vi "RHRT-IGVC-2013.vi"() -> ()   [LabVIEW 2012]
doc: "This the Rose-Hulman Robotics Tream IGVC compatition Code\nexample demonstrates the control of an autonomous robot through multiple asynchronous processes, modeled by VIs, that communicate with each other using shared variables. This example also shows an obstacle avoidance algorithm that the simulated robot uses as it navigates. The application includes the following processes:\n\n1. LIDAR Loop (\"Sense\")--Uses LabVIEW dataflow programming to generate simulated sensor data based on the position of the robot and any obstacles in the environment.\n\n2. Operator Loop (\"Think\")--Uses a state machine to control the movement of the robot according to commands from the user. When the robot follows a path without joystick or keyboard control, this process controls the attitude of the autonomous robot using a Vector Field Histogram (VFH) algorithm to avoid obstacles.\n\n3. Motor Loop (\"Act\")--Uses a Control and Simulation Loop, from the Control Design and Simulation Module, to create a model of the robot, simulate its dynamic behavior, and show the control loops and attitude observers."
uses:
  <vilib>/robotics/Controls/Compass Indicator/Compass Indicator.xctl
  <vilib>/Platform/TimedLoop/XDataNode/timing_clust.ctl
  <vilib>/Platform/TimedLoop/XDataNode/nitl_modes.ctl
  <vilib>/Platform/TimedLoop/XDataNode/wakeup.ctl
  <vilib>/Platform/TimedLoop/XDataNode/XDataNode.xnode
  <vilib>/Platform/TimedLoop/XDataNode/XDNodeRunTimeDep.lvlib
panel:
  out "Robot Model":u16
  in  "Robot Model:":T1(ring)
  out "Error":bool
  out "OK":bool
  in  "HUD 2":enum32{"GPS", "LIDAR", "IMU", "Occupancy Grid"}(tab)
  out "Health":u8(slide) scale=0.0..12.0
  out "XY Graph 2":cluster{dbl[], dbl[]}(graph)
  out "Data Aquired 2":picture
  out "Digree 2":dbl=16.3201904296875 caption="Digree"
  out "Compass Indicator 2":dbl(xcontrol)=16.3201904296875
  out "Occupancy Grid":dbl[][](graph)
  in  "Telemetry":T2(tab)
  out "Voltage":cluster{sgl, sgl, sgl}(knob)={13.4, 12.0, 47.48} caption="Main Battery Voltage\nInternal Voltage\nDSUB Voltage" scale=8.0..15.0
  out "Current":cluster{sgl, sgl, sgl, sgl}(knob)={0.0, 0.0, -2.0, -2.0} caption="Ch1 Motor Curret\nCh2 Motor Curret\nCh1 Battery Curret \nCh2 Battery Curret" scale=0.0..15.0
  out "IC Temp (C)":i32(slide)=22 scale=0.0..150.0
  out "Ch1 Temp (C)":i32(slide)=22 scale=0.0..150.0
  out "Ch2 Temp (C)":i32(slide)=23 scale=0.0..150.0
  out "Ch1 Encoder Speed\nCh2 Encoder Speed":cluster{i32, i32}(knob) scale=-300.0..300.0
  out "Image Out":T3(plugin-control)
  in  "Search For VISA":bool
  in  "HUD":T4(tab)=enum."Info"
  in  "Analog Stick":cluster{dbl, dbl}[](graph)
  in  "Clear Breadcrumbs":bool
  in  "Max Points":dbl=3000.0 format="%0.2f"
  out "XY Graph":cluster{dbl[], dbl[]}[](graph)
  out "Longitude Point":dbl format="%#_12g"
  out "Latitude Point":dbl format="%#_12g"
  out "Data Aquired":picture
  in  "Max Distance":dbl=3000.0 format="%0.2f"
  out "Digree":dbl=16.3201904296875
  out "Compass Indicator":dbl(xcontrol)=16.3201904296875
  out "Curretn POI":string
  in  "Curent Index":i32
  in  "Waypoint Table":string[][](table)=[["1.000000", "39.400000", "-87.200000"], ["2.000000", "39.600000", "-87.300000"], ["2.000000", "39.200000", "-87.400000"]]
  in  "Show GPS Diagram":bool
  in  "Show LL Diagram":bool
  in  "Show AI Diagram":bool
  in  "Show MCL Diagram":bool
  in  "About":bool
  in  "Stop":bool
  in  "Error Display":T5(tab)
  out "Cammera Status":bool
  out "Cammera Status 2":bool
  out "IMU Status":bool
  in  "IMU VISA":refnum<visa-resource-name>="COM7"
  out "Motor Status":bool
  in  "Motor VISA":refnum<visa-resource-name>="COM21"
  out "LIDAR Status":bool
  in  "LIDAR VISA":refnum<visa-resource-name>="COM20"
  out "GPS Status":bool
  in  "GPS VISA":refnum<visa-resource-name>="COM22"
  in  "GPS Error":errorcluster
  in  "LIDAR Error":errorcluster
  in  "Motor Error":errorcluster
  in  "IMU Error":errorcluster
  in  "Camera Error":errorcluster
  in  "Robot Mode:":T6(ring)
  out "End Loop":bool=TRUE
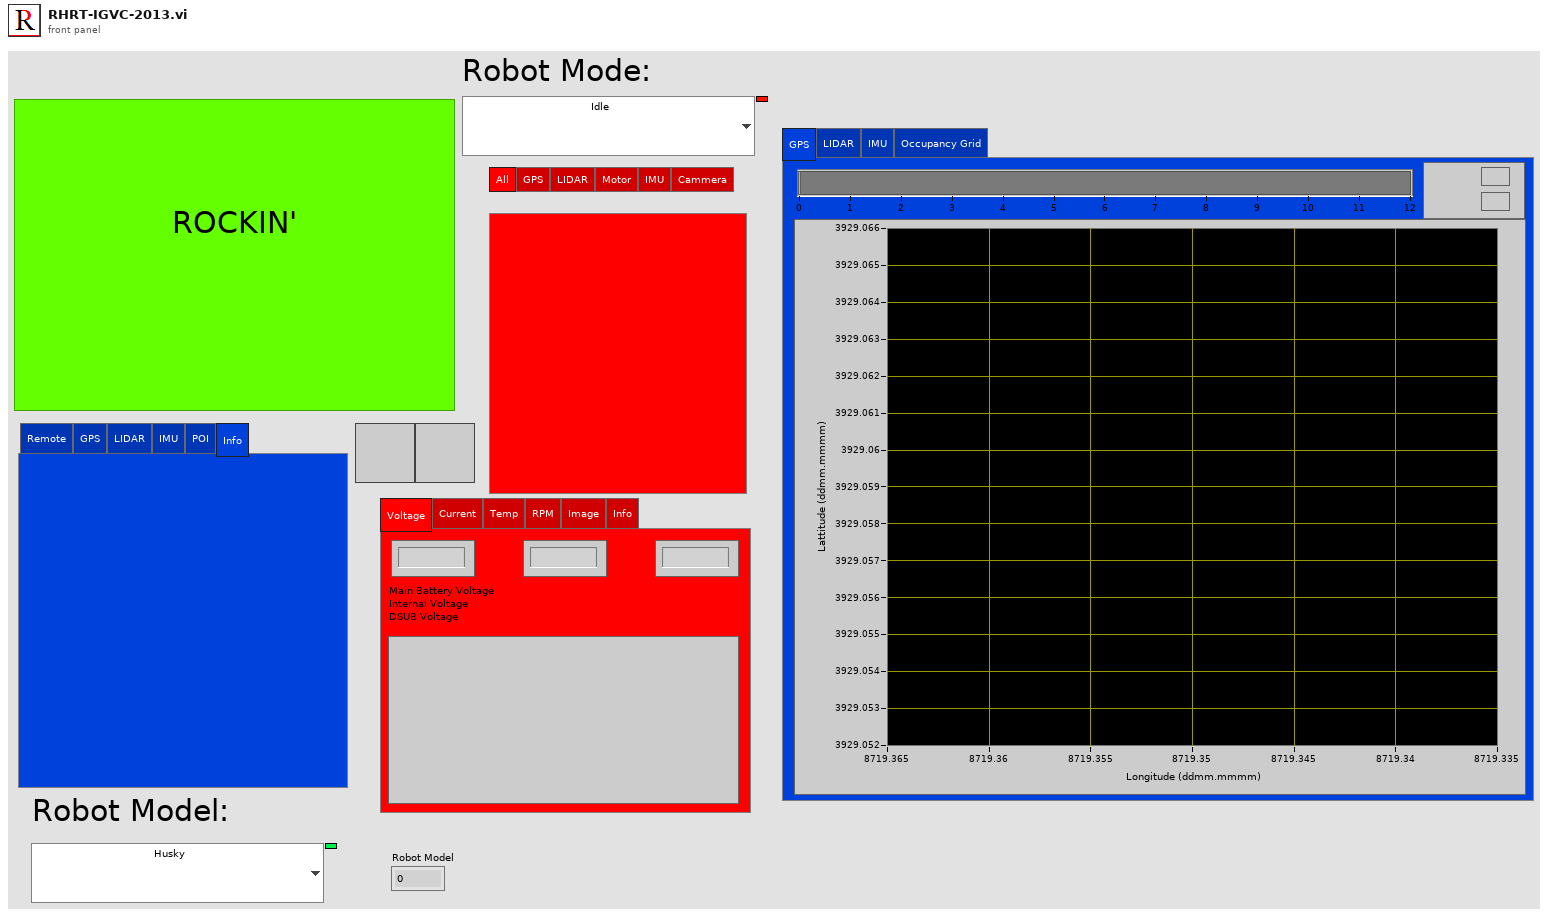
[diagram p1: front panel]
types:
  T1 = enum16{"Husky", "Galatea", "Sim Husky", "Sim Galatea"}
  T2 = enum32{"Voltage", "Current", "Temp", "RPM", "Image", "Info"}
  T3 = typedef "IMAQ Image.ctl" = refnum<image>
  T4 = enum32{"Remote", "GPS", "LIDAR", "IMU", "POI", "Info"}
  T5 = enum32{"All", "GPS", "LIDAR", "Motor", "IMU", "Cammera"}
  T6 = enum16{"Idle", "Wiimote", "Joypad", "IGVC", "Avoide Objects", "Avoide Lines", "Path Planning", "Heading", "Waypoint"}
  T7 = typedef "XDNodeRunTimeDep.lvlib/timing_clust.ctl" = cluster{"Expected End [f-1]":u64, "Actual End [f-1]":u64, "Finished Late? [f-1]":bool, "Expected End [i-1]":u64, "Actual End [i-1]":u64, "Finished Late? [i-1]":bool, "Expected Start [i]":u64, "Actual Start [i]":u64, "Expected Start [f]":u64, "Actual Start [f]":u64, "Source Name":string, "Structure Name":string, "Period":i64, "Deadline":i64, "Offset":i64, "Start":i64, "Priority":i32, "Timeout":i32, "Mode":T8, "Wakeup Reason":T9, "Error":errorcluster, "Source Type":string, "Secondary Source Type":string, "Global End Time":u64, "Global Start Time":u64, "Frame Duration":u64, "Iteration Duration":u64, "Assigned CPU":i32, "I/O Scan Engine Mode":u32}
  T8 = typedef "XDNodeRunTimeDep.lvlib/nitl_modes.ctl" = enum32{"No Change", "Process missed periods, maintain original phase", "Discard missed periods, maintain original phase", "Process missed periods, ignore original phase", "Discard missed periods, ignore original phase"}
  T9 = typedef "XDNodeRunTimeDep.lvlib/wakeup.ctl" = enum32{"Normal", "Aborted", "Asynchronous wakeup", "Timing source error", "Timed loop error", "Timeout"}
  T10 = cluster{"Latitude":dbl, "Longitude":dbl, "Altitude":dbl, "Velocity, Correction & SET":cluster{"Velocity North":dbl, "Velocity East":dbl, "Velocity Up":dbl, "Ellipsoidal Height":dbl, "GDOP":sgl, "PDOP":sgl, "HDOP":sgl, "VDOP":sgl, "TDOP":sgl, "Horizontal Figure of Merit":u8, "Time Figure of Merit":u8, "Max dGPS Age":sgl, "Extended Navigation Mode":u8, "Antenna Height Adjustment ":dbl, "SET North":i32, "SET East":i32, "SET Up":i32}, "Time":cluster{"GPS Week":u16, "GPS Time of Week":sgl}, "Satellites Used":i32[]}
  T11 = cluster{"Azimuth":dbl, "FocusPointAltitude":dbl, "altMode":i32, "FocusPointLatitude":dbl, "FocusPointLongitude":dbl, "Range":dbl, "Tilt":dbl}
  T12 = cluster{"Position":cluster{"Roll":dbl, "Pitch":dbl, "Yaw":dbl}, "Orientation Matrix":dbl[][], "Magnetic Field":cluster{"Z-Axis Magnetic Field":dbl, "Y-Axis Magnetic Field":dbl, "X-Axis Magnetic Field":dbl}, "Acceleration":cluster{"Z-Axis Acceleration":dbl, "Y-Axis Acceleration":dbl, "X-Axis Acceleration":dbl}, "Angular Rate":cluster{"X-Axis Angular Rate":dbl, "Y-Axis Angular Rate":dbl, "Z-Axis Angular Rate":dbl}, "Quaternion":dbl[]}
  T13 = cluster{"Voltage":cluster{sgl, sgl, sgl}, "Encoder Speed":cluster{i32, i32}, "Temps":cluster{"IC Temp (C)":i32, "Ch1 Temp (C)":i32, "Ch2 Temp (C)":i32}, "Current":cluster{dbl, dbl, dbl, dbl}}
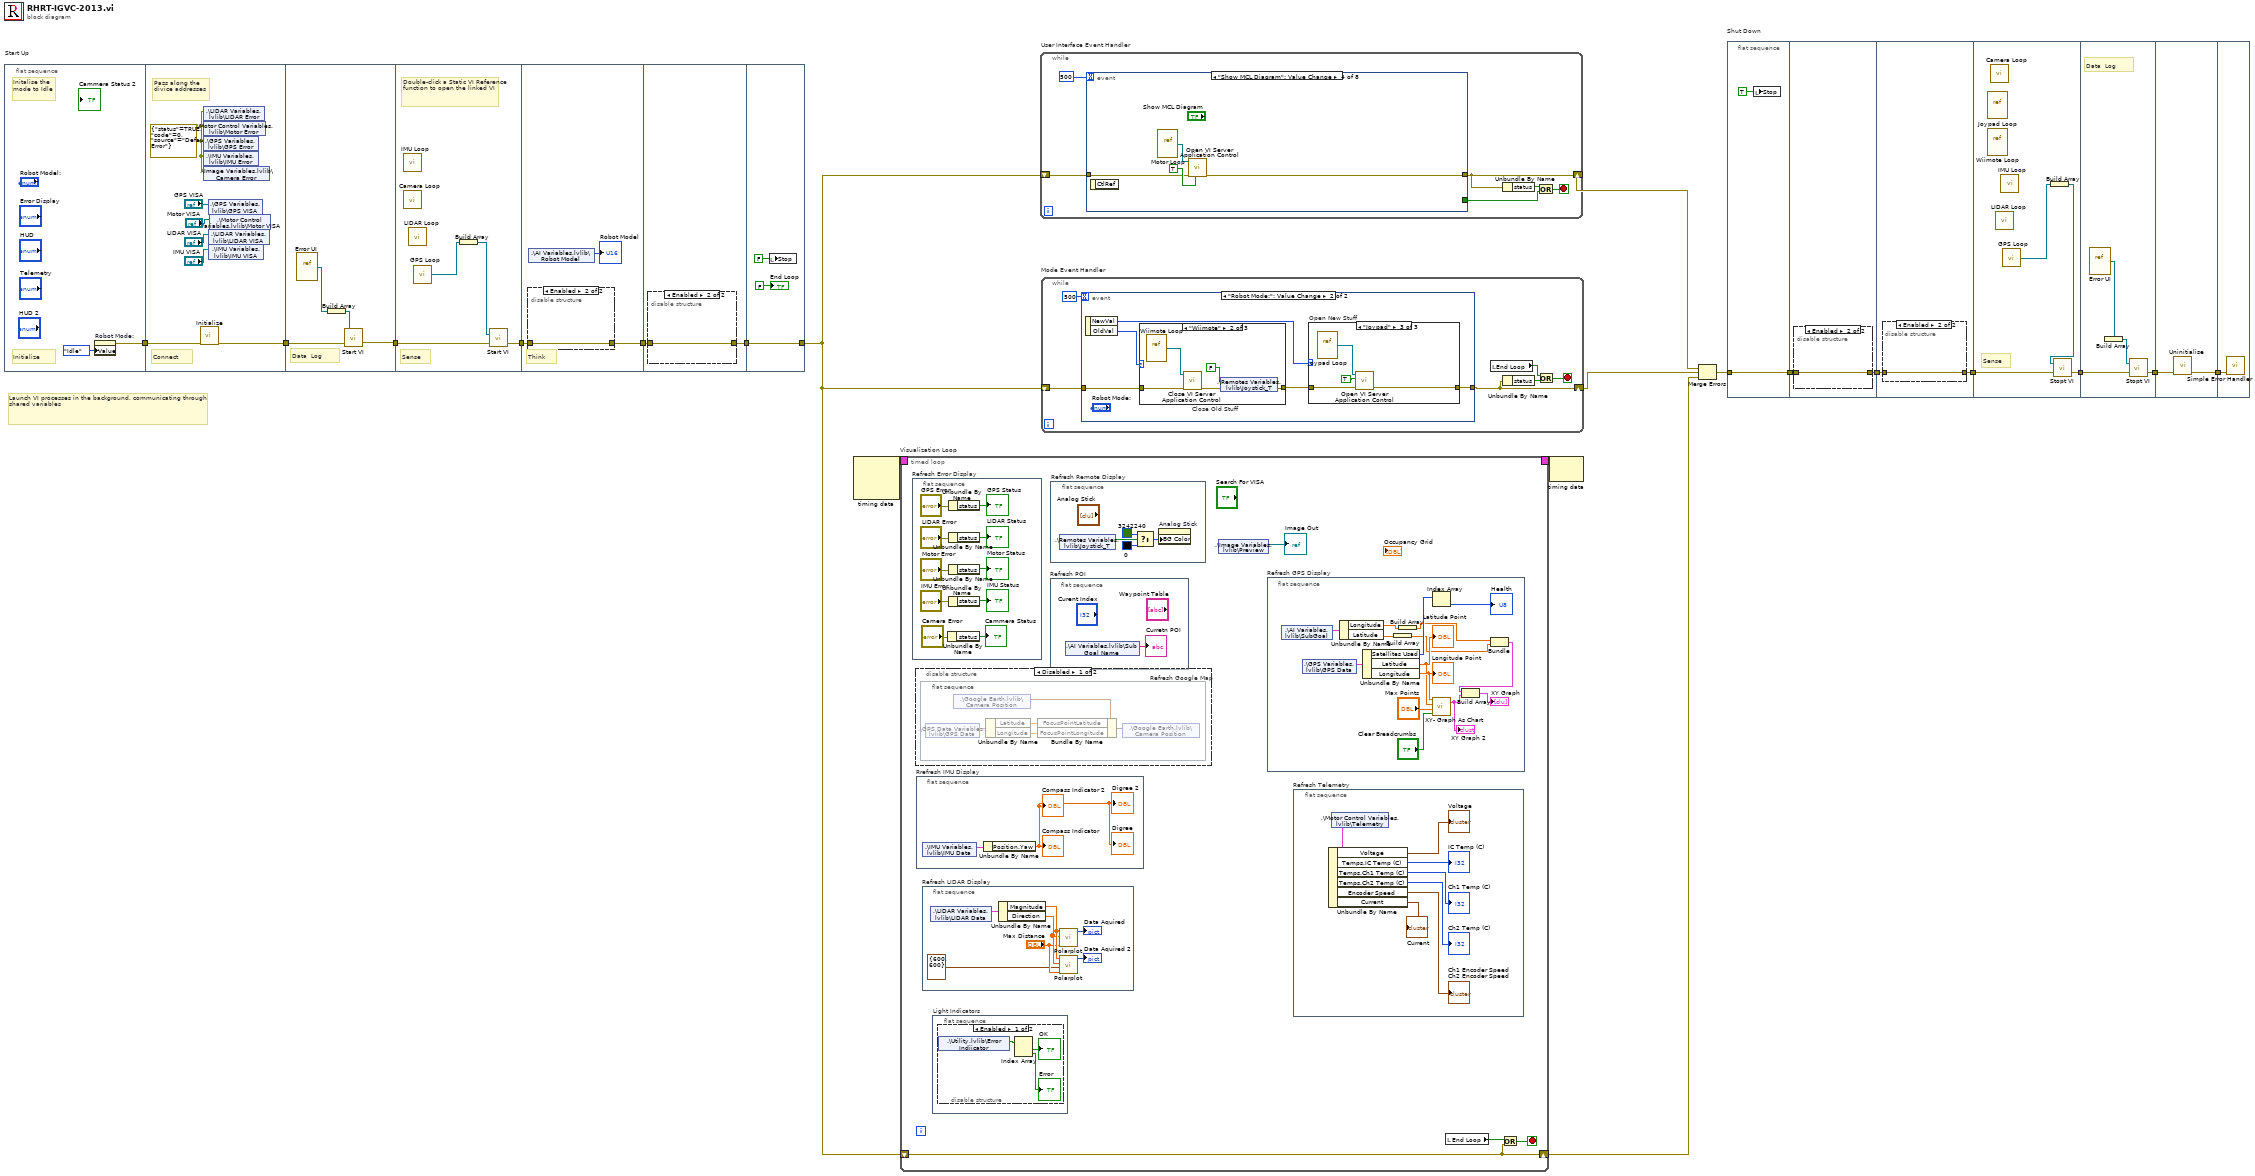
[diagram p0: block diagram]
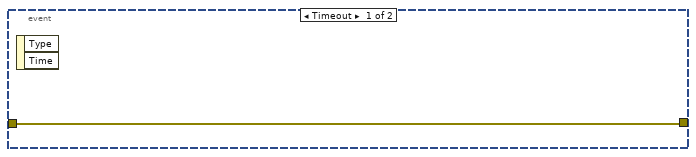
[diagram p2: hidden frame]
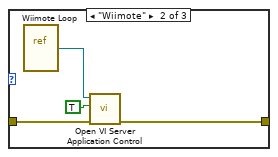
[diagram p4: hidden frame]
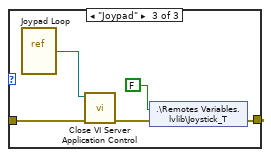
[diagram p6: hidden frame]
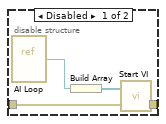
[diagram p7: hidden frame]
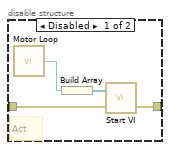
[diagram p8: hidden frame]
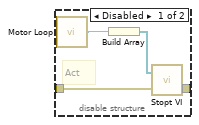
[diagram p9: hidden frame]
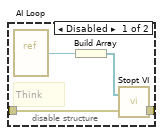
[diagram p10: hidden frame]
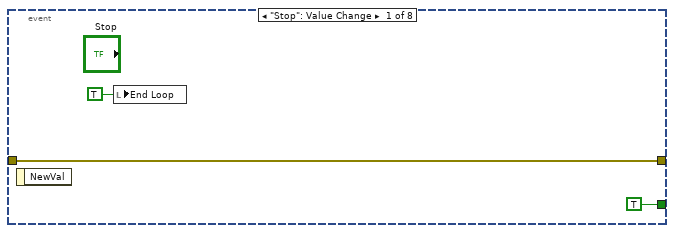
[diagram p11: hidden frame]
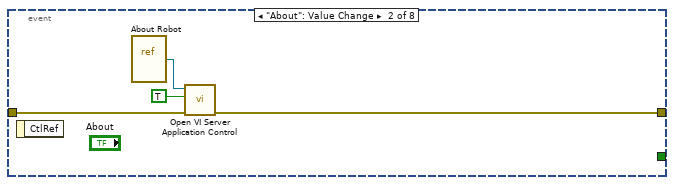
[diagram p12: hidden frame]
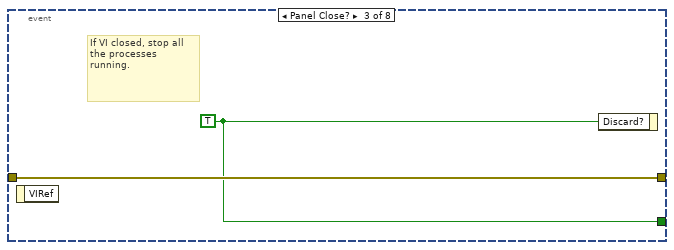
[diagram p13: hidden frame]
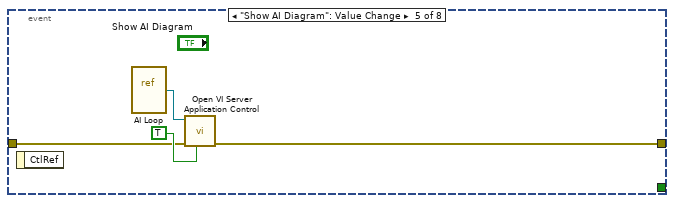
[diagram p14: hidden frame]
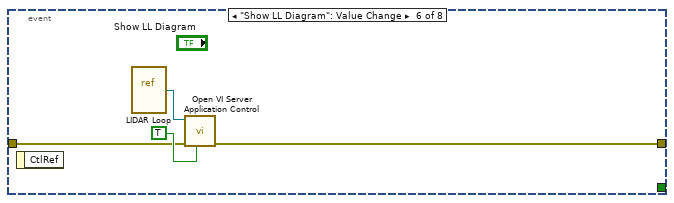
[diagram p15: hidden frame]
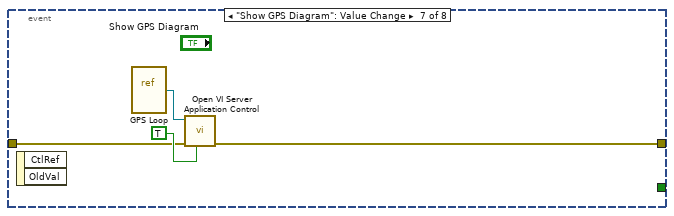
[diagram p16: hidden frame]
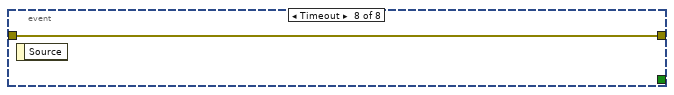
[diagram p17: hidden frame]
diagram:
  # "Launch VI processes in the background, communicating through shared variables"
  n1 = flat-sequence "Start Up" {
    tunnel: [w21] -> w14
    tunnel: [w22] -> w6
    tunnel: w14 -> [w23]
    tunnel: w6 -> [w32]
    tunnel: [w31] -> w3
    tunnel: [w34] -> w13
    tunnel: w3 -> [w35]
    tunnel: w13 -> [w39]
    tunnel: [w38] -> w11
    tunnel: [w45] -> w12
    tunnel: w11 -> [w46]
    tunnel: [w54] -> w7
    tunnel: w12 -> [w54]
    frame #0 {
      # "Initialize"
      # "Initalise the mode to Idle"
      n2 = property on="Robot Mode:" class="Enum (strict)"("Value"=T6."Idle" ("Robot Mode:")) -> (error out=w21:errorcluster)  [unwired: 2 in, 1 out]
    }
    frame #1 {
      w24 = errorcluster {"status"=TRUE, "code"=0, "source"="Default Error"} ("error out")
      # "Connect"
      # "Pass along the divice addresses"
      n3 = call "Initialize.vi"("Error In"=w23) -> ("Error Out"=w22:errorcluster)  [unwired: 10 in]
      n4 = shared-variable ".\\LIDAR Variables.lvlib\\LIDAR Error"(w24) -> ()  [unwired: 1 in, 1 out]
      n5 = shared-variable ".\\Motor Control Variables.lvlib\\Motor Error"(w24) -> ()  [unwired: 1 in, 1 out]
      n6 = shared-variable ".\\GPS Variables.lvlib\\GPS Error"(w24) -> ()  [unwired: 1 in, 1 out]
      n7 = shared-variable ".\\IMU Variables.lvlib\\IMU Error"(w24) -> ()  [unwired: 1 in, 1 out]
      n8 = shared-variable ".\\Image Variables.lvlib\\Camera Error"(w24) -> ()  [unwired: 1 in, 1 out]
      n9 = shared-variable ".\\GPS Variables.lvlib\\GPS VISA"("GPS VISA") -> ()  [unwired: 1 in, 1 out]
      n10 = shared-variable ".\\LIDAR Variables.lvlib\\LIDAR VISA"("LIDAR VISA") -> ()  [unwired: 1 in, 1 out]
      n11 = shared-variable ".\\IMU Variables.lvlib\\IMU VISA"("IMU VISA") -> ()  [unwired: 1 in, 1 out]
      n12 = shared-variable ".\\Motor Control Variables.lvlib\\Motor VISA"("Motor VISA") -> ()  [unwired: 1 in, 1 out]
    }
    frame #2 {
      # "Data  Log"
      n13 = vi-ref "Error UI.vi"() -> (w29:refnum<vi>)
      n14 = Build Array(w29) -> (w30:refnum<vi>[])
      n15 = call "Start VI.vi"("error in"=w32, "VI refnum"=w30) -> ("error out"=w31:errorcluster)  [unwired: 1 in]
    }
    frame #3 {
      # "Double-click a Static VI Reference function to open the linked VI"
      # "Sense"
      n16 = call "IMU Loop.vi"() -> ()  [unwired: 1 in, 1 out]
      n17 = call "Camera Loop.vi"() -> ()  [unwired: 1 in, 1 out]
      n18 = call "LIDAR Loop.vi"() -> ()  [unwired: 1 in, 1 out]
      n19 = call "GPS Loop.vi"() -> ("VI Refnum"=w33:refnum<vi>)  [unwired: 1 in]
      n20 = Build Array(w33) -> (w36:refnum<vi>[])
      n21 = call "Start VI.vi"("error in"=w35, "VI refnum"=w36) -> ("error out"=w34:errorcluster)  [unwired: 1 in]
    }
    frame #4 {
      # "Think"
      n22 = disable-structure shown="Enabled" {
        disable-tunnel: w39 -> [w43 w44]
        disable-tunnel: [w42 w44] -> w38
        frame Disabled {
          n23 = vi-ref "AI Loop.vi"() -> (w41:refnum<vi>)
          n24 = Build Array(w41) -> (w40:refnum<vi>[])
          n25 = call "Start VI.vi"("error in"=w43, "VI refnum"=w40) -> ("error out"=w42:errorcluster)  [unwired: 1 in]
        }
        frame Enabled {
        }
      }
      n26 = shared-variable ".\\AI Variables.lvlib\\Robot Model"() -> (→"Robot Model":u16)  [unwired: 1 in, 1 out]
    }
    frame #5 {
      n27 = disable-structure shown="Enabled" {
        disable-tunnel: w46 -> [w50 w51]
        disable-tunnel: [w49 w51] -> w45
        frame Disabled {
          # "Act"
          n28 = call "Motor Loop.vi"() -> ("VI Refnum"=w47:refnum<vi>)  [unwired: 1 in]
          n29 = Build Array(w47) -> (w48:refnum<vi>[])
          n30 = call "Start VI.vi"("error in"=w50, "VI refnum"=w48) -> ("error out"=w49:errorcluster)  [unwired: 1 in]
        }
        frame Enabled {
        }
      }
    }
    frame #6 {
      n31 = local write "Stop"(FALSE ("Halt TL")) -> ()
      "End Loop" <- FALSE ("Halt TL")
    }
  }
  n32 = node-c288() -> (w19:T7)  [unwired: 3 in]
  n33 = timed-loop "Visualization Loop" {
    timing: w19 -> [_]
    timing-out: [_] -> w18
    shift-right: [w55] -> w4
    shift-left: w7 -> [w55]
    stop <- w58 stop-if-true
    n34 = flat-sequence "Refresh Error Display" {
      frame #0 {
        n35 = Unbundle By Name("Camera Error") -> ("status"=→"Cammera Status":bool)
        n36 = Unbundle By Name("GPS Error") -> ("status"=→"GPS Status":bool)
        n37 = Unbundle By Name("LIDAR Error") -> ("status"=→"LIDAR Status":bool)
        n38 = Unbundle By Name("Motor Error") -> ("status"=→"Motor Status":bool)
        n39 = Unbundle By Name("IMU Error") -> ("status"=→"IMU Status":bool)
      }
    }
    n40 = disable-structure shown="Disabled" {
      frame Disabled {
        n41 = flat-sequence "Refresh Google Map" {
          frame #0 {
            n42 = shared-variable ".\\GPS Data Variables.lvlib\\GPS Data"() -> (w62:T10)  [unwired: 1 in, 1 out]
            n43 = shared-variable ".\\Google Earth.lvlib\\Camera Position"() -> (w63:T11)  [unwired: 1 in, 1 out]
            n44 = Unbundle By Name(w62) -> ("Latitude"=w59:dbl, "Longitude"=w61:dbl)
            n45 = Bundle By Name(cluster=w63, "FocusPointLatitude"=w59, "FocusPointLongitude"=w61) -> (w60:T11)
            n46 = shared-variable ".\\Google Earth.lvlib\\Camera Position"(w60) -> ()  [unwired: 1 in, 1 out]
          }
        }
      }
      frame Enabled {
      }
    }
    n47 = flat-sequence "Rrefresh IMU Display" {
      frame #0 {
        n48 = shared-variable ".\\IMU Variables.lvlib\\IMU Data"() -> (w91:T12)  [unwired: 1 in, 1 out]
        n49 = Unbundle By Name(w91) -> ("Position.Yaw"=→"Compass Indicator" →"Digree" →"Compass Indicator 2" →"Digree 2":dbl)
      }
    }
    n50 = flat-sequence "Refresh LIDAR Display" {
      frame #0 {
        n51 = shared-variable ".\\LIDAR Variables.lvlib\\LIDAR Data"() -> (w73:cluster{"Magnitude":dbl[], "Direction":dbl[]})  [unwired: 1 in, 1 out]
        n52 = Unbundle By Name(w73) -> ("Magnitude"=w70:dbl[], "Direction"=w69:dbl[])
        n53 = call "Polarplot.vi"("maximum"="Max Distance", "Direction"=w69, "Magnitude"=w70) -> ("Data Aquired"=→"Data Aquired":picture)  [unwired: 8 in]
        n54 = call "Polarplot.vi"("maximum"="Max Distance", "dimensions (w,h)"=cluster{"width":i16, "height":i16} {"width"=600, "height"=600}, "Direction"=w69, "Magnitude"=w70) -> ("Data Aquired"=→"Data Aquired 2":picture)  [unwired: 7 in]
      }
    }
    n55 = flat-sequence "Light Indicators" {
      frame #0 {
        n56 = disable-structure shown="Enabled" {
          frame Enabled {
            n57 = shared-variable ".\\Utility.lvlib\\Error Indiicator"() -> (w66:bool[])  [unwired: 1 in, 1 out]
            n58 = Index Array(array=w66) -> (element #1=→"OK":bool, element #2=→"Error":bool)  [unwired: 2 in]
          }
          frame Disabled {
          }
        }
      }
    }
    n59 = flat-sequence "Refresh POI" {
      frame #0 {
        n60 = shared-variable ".\\AI Variables.lvlib\\Sub Goal Name"() -> (→"Curretn POI":string)  [unwired: 1 in, 1 out]
      }
    }
    n61 = flat-sequence "Refresh Remote Display" {
      frame #0 {
        n62 = shared-variable ".\\Remotes Variables.lvlib\\Joystick_T"() -> (w100:bool)  [unwired: 1 in, 1 out]
        n63 = Select(t=u32 3242240, s=w100, f=u32 0) -> (s? t:f=w99:u32)
        n64 = property on="Analog Stick" class="XYGraph (strict)"("BG Color"=w99) -> ()  [unwired: 2 in, 2 out]
      }
    }
    n65 = shared-variable ".\\Image Variables.lvlib\\Preview"() -> (→"Image Out":refnum<image>)  [unwired: 1 in, 1 out]
    n66 = flat-sequence "Refresh GPS Display" {
      frame #0 {
        n67 = shared-variable ".\\AI Variables.lvlib\\SubGoal"() -> (w84:T10)  [unwired: 1 in, 1 out]
        n68 = shared-variable ".\\GPS Variables.lvlib\\GPS Data"() -> (w88:T10)  [unwired: 1 in, 1 out]
        n69 = Unbundle By Name(w84) -> ("Longitude"=w79:dbl, "Latitude"=w78:dbl)
        n70 = Unbundle By Name(w88) -> ("Satellites Used"=w85:i32[], "Latitude"=w82:dbl, "Longitude"=w83:dbl)
        "Latitude Point" <- w82
        "Longitude Point" <- w83
        n71 = Build Array(w78) -> (w76:dbl[])
        n72 = Build Array(w79) -> (w77:dbl[])
        n73 = Index Array(array=w85) -> (element=→"Health":i32)  [unwired: 1 in]
        n74 = call "XY- Graph As Chart.vi"("Clear Graph (F)"="Clear Breadcrumbs", "Maxi Points (10,000)"="Max Points", "Y-Value"=w82, "X- Value"=w83) -> ("XY Graph"=w81:cluster{dbl[], dbl[]})  [unwired: 1 out]
        "XY Graph 2" <- w81
        n75 = Bundle(w77, w76) -> (w75:cluster{dbl[], dbl[]})  [unwired: 1 out]
        n76 = Build Array(w75, w81) -> (→"XY Graph":cluster{dbl[], dbl[]}[])
      }
    }
    n77 = flat-sequence "Refresh Telemetry" {
      frame #0 {
        n78 = shared-variable ".\\Motor Control Variables.lvlib\\Telemetry"() -> (w98:T13)  [unwired: 1 in, 1 out]
        n79 = Unbundle By Name(w98) -> ("Voltage"=→"Voltage":cluster{sgl, sgl, sgl}, "Temps.IC Temp (C)"=→"IC Temp (C)":i32, "Temps.Ch1 Temp (C)"=→"Ch1 Temp (C)":i32, "Temps.Ch2 Temp (C)"=→"Ch2 Temp (C)":i32, "Encoder Speed"=→"Ch1 Encoder Speed\nCh2 Encoder Speed":cluster{i32, i32}, "Current"=→"Current":cluster{dbl, dbl, dbl, dbl})
      }
    }
    n80 = local read "End Loop"() -> (w56:bool)
    n81 = Or(x=w56, y=w55) -> (x .or. y?=w58:bool)
  }
  n82 = while "User Interface Event Handler" {
    shift-right: [w117] -> w17
    shift-left: w7 -> [w120]
    stop <- w119 stop-if-true
    n83 = event shown="[3] \"Show MCL Diagram\": Value Change" {
      selector: _ -> [_ _ _ _ _ _ _ _]
      dyn-events: _ -> [_ _ _ _ _ _ _ _]
      timeout: 500 -> [_ _ _ _ _ _ _ _]
      tunnel: [TRUE _ w128 _ _ _ _ _] -> w115
      tunnel: w120 -> [w123 w126 w129 w131 w135 w139 w142 w146]
      tunnel: [w123 w125 w129 w130 w134 w138 w143 w146] -> w117
      event "Stop": Value Change {
        n84 = event-data() -> ()  [unwired: 2 out]
        n85 = local write "End Loop"(TRUE ("End Loop")) -> ()
      }
      event "About": Value Change {
        n86 = event-data() -> ()  [unwired: 2 out]
        n87 = vi-ref "About Robot.vi"() -> (w127:refnum<vi>)
        n88 = call "Open VI Server Application Control.vi"("error in (no error)"=w126, "run VI (F)"=TRUE ("Launch Map"), "VI refnum"=w127) -> ("error out"=w125:errorcluster)  [unwired: 8 in]
      }
      event Panel Close? {
        w128 = TRUE ("Discard?")
        # "If VI closed, stop all the processes running."
        n89 = event-data() -> ()  [unwired: 2 out]
        n90 = event-data("Discard?"=w128) -> ()  [unwired: 1 in, 1 out]
      }
      event "Show MCL Diagram": Value Change {
        n91 = event-data() -> ()  [unwired: 2 out]
        n92 = vi-ref "Motor Loop.vi"() -> (w133:refnum<vi>)
        n93 = call "Open VI Server Application Control.vi"("open block diagram (F)"=TRUE ("Open Front Panel"), "error in (no error)"=w131, "VI refnum"=w133) -> ("error out"=w130:errorcluster)  [unwired: 8 in]
      }
      event "Show AI Diagram": Value Change {
        n94 = event-data() -> ()  [unwired: 2 out]
        n95 = vi-ref "AI Loop.vi"() -> (w136:refnum<vi>)
        n96 = call "Open VI Server Application Control.vi"("open block diagram (F)"=TRUE ("Open Front Panel"), "error in (no error)"=w135, "VI refnum"=w136) -> ("error out"=w134:errorcluster)  [unwired: 8 in]
      }
      event "Show LL Diagram": Value Change {
        n97 = event-data() -> ()  [unwired: 2 out]
        n98 = vi-ref "LIDAR Loop.vi"() -> (w140:refnum<vi>)
        n99 = call "Open VI Server Application Control.vi"("open block diagram (F)"=TRUE ("Open Front Panel"), "error in (no error)"=w139, "VI refnum"=w140) -> ("error out"=w138:errorcluster)  [unwired: 8 in]
      }
      event "Show GPS Diagram": Value Change {
        n100 = event-data() -> ()  [unwired: 3 out]
        n101 = vi-ref "GPS Loop.vi"() -> (w144:refnum<vi>)
        n102 = call "Open VI Server Application Control.vi"("open block diagram (F)"=TRUE ("Open Front Panel"), "error in (no error)"=w142, "VI refnum"=w144) -> ("error out"=w143:errorcluster)  [unwired: 8 in]
      }
      event Timeout {
        n103 = event-data() -> ()  [unwired: 2 out]
      }
    }
    n104 = Unbundle By Name(w117) -> ("status"=w116:bool)
    n105 = Or(x=w116, y=w115) -> (x .or. y?=w119:bool)
  }
  n106 = while "Mode Event Handler" {
    shift-right: [w149] -> w8
    shift-left: w7 -> [w150]
    stop <- w151 stop-if-true
    n107 = event shown="[1] \"Robot Mode:\": Value Change" {
      selector: _ -> [_ _]
      dyn-events: _ -> [_ _]
      timeout: 500 -> [_ _]
      tunnel: [w153 w156] -> w149
      tunnel: w150 -> [w153 w158]
      event Timeout {
        n108 = event-data() -> ()  [unwired: 1 in, 2 out]
      }
      event "Robot Mode:": Value Change {
        n109 = event-data() -> ("NewVal"=w155:T6, "OldVal"=w154:T6)  [unwired: 1 in]
        n110 = case "Close Old Stuff" shown="\"Wiimote\"" w154 {
          tunnel: w158 -> [w168 w173 w178]
          tunnel: [w168 w169 w174] -> w157
          frame "Idle", Default {
          }
          frame "Wiimote" {
            n111 = vi-ref "Wiimote Loop.vi"() -> (w172:refnum<vi>)
            n112 = call "Close VI Server Application Control.vi"("error in (no error)"=w173, "VI refnum"=w172) -> ("error out"=w170:errorcluster)  [unwired: 9 in]
            n113 = shared-variable ".\\Remotes Variables.lvlib\\Joystick_T"(FALSE ("Joystick_T"), error in=w170) -> (error out=w169:errorcluster)
          }
          frame "Joypad" {
            n114 = vi-ref "Joypad Loop.vi"() -> (w177:refnum<vi>)
            n115 = call "Close VI Server Application Control.vi"("error in (no error)"=w178, "VI refnum"=w177) -> ("error out"=w175:errorcluster)  [unwired: 9 in]
            n116 = shared-variable ".\\Remotes Variables.lvlib\\Joystick_T"(FALSE ("Joystick_T"), error in=w175) -> (error out=w174:errorcluster)
          }
        }
        n117 = case "Open New Stuff" shown="\"Joypad\"" w155 {
          tunnel: w157 -> [w159 w163 w167]
          tunnel: [w159 w161 w165] -> w156
          frame "Idle", Default {
          }
          frame "Wiimote" {
            n118 = vi-ref "Wiimote Loop.vi"() -> (w160:refnum<vi>)
            n119 = call "Open VI Server Application Control.vi"("error in (no error)"=w163, "run VI (F)"=TRUE, "VI refnum"=w160) -> ("error out"=w161:errorcluster)  [unwired: 8 in]
          }
          frame "Joypad" {
            n120 = vi-ref "Joypad Loop.vi"() -> (w164:refnum<vi>)
            n121 = call "Open VI Server Application Control.vi"("error in (no error)"=w167, "run VI (F)"=TRUE, "VI refnum"=w164) -> ("error out"=w165:errorcluster)  [unwired: 8 in]
          }
        }
      }
    }
    n122 = local read "End Loop"() -> (w148:bool)
    n123 = Unbundle By Name(w149) -> ("status"=w152:bool)
    n124 = Or(x=w148, y=w152) -> (x .or. y?=w151:bool)
  }
  n125 = node-c288(w18) -> ()  [unwired: 1 out]
  n126 = Merge Errors(w17, w8, w4) -> (w15:errorcluster)
  n127 = flat-sequence "Shut Down" {
    tunnel: w15 -> [w179]
    tunnel: [w179] -> w16
    tunnel: w16 -> [w182]
    tunnel: [w181] -> w10
    tunnel: w10 -> [w189]
    tunnel: [w188] -> w9
    tunnel: w9 -> [w198]
    tunnel: [w197] -> w5
    tunnel: w5 -> [w200]
    tunnel: [w202] -> w2
    tunnel: w2 -> [w204]
    tunnel: [w203] -> w1
    tunnel: w1 -> [w205]
    frame #0 {
      n128 = local write "Stop"(TRUE ("Halt TL")) -> ()
    }
    frame #1 {
      n129 = disable-structure shown="Enabled" {
        disable-tunnel: w182 -> [w186 w187]
        disable-tunnel: [w185 w187] -> w181
        frame Disabled {
          # "Act"
          n130 = call "Motor Loop.vi"() -> ("VI Refnum"=w183:refnum<vi>)  [unwired: 1 in]
          n131 = Build Array(w183) -> (w184:refnum<vi>[])
          n132 = call "Stopt VI.vi"("error in"=w186, "VI refnum"=w184) -> ("error out"=w185:errorcluster)  [unwired: 1 in]
        }
        frame Enabled {
        }
      }
    }
    frame #2 {
      n133 = disable-structure shown="Enabled" {
        disable-tunnel: w189 -> [w193 w194]
        disable-tunnel: [w192 w194] -> w188
        frame Disabled {
          # "Think"
          n134 = vi-ref "AI Loop.vi"() -> (w190:refnum<vi>)
          n135 = Build Array(w190) -> (w191:refnum<vi>[])
          n136 = call "Stopt VI.vi"("error in"=w193, "VI refnum"=w191) -> ("error out"=w192:errorcluster)  [unwired: 1 in]
        }
        frame Enabled {
        }
      }
    }
    frame #3 {
      # "Sense"
      n137 = vi-ref "Joypad Loop.vi"() -> ()  [unwired: 1 out]
      n138 = vi-ref "Wiimote Loop.vi"() -> ()  [unwired: 1 out]
      n139 = call "Camera Loop.vi"() -> ()  [unwired: 1 in, 1 out]
      n140 = call "LIDAR Loop.vi"() -> ()  [unwired: 1 in, 1 out]
      n141 = call "IMU Loop.vi"() -> ()  [unwired: 1 in, 1 out]
      n142 = call "GPS Loop.vi"() -> ("VI Refnum"=w195:refnum<vi>)  [unwired: 1 in]
      n143 = Build Array(w195) -> (w196:refnum<vi>[])
      n144 = call "Stopt VI.vi"("error in"=w198, "VI refnum"=w196) -> ("error out"=w197:errorcluster)  [unwired: 1 in]
    }
    frame #4 {
      # "Data  Log"
      n145 = vi-ref "Error UI.vi"() -> (w199:refnum<vi>)
      n146 = Build Array(w199) -> (w201:refnum<vi>[])
      n147 = call "Stopt VI.vi"("error in"=w200, "VI refnum"=w201) -> ("error out"=w202:errorcluster)  [unwired: 1 in]
    }
    frame #5 {
      n148 = call "Uninitialise.vi"("Error In"=w204) -> ("Error Out"=w203:errorcluster)  [unwired: 10 in]
    }
    frame #6 {
      n149 = call <vilib>:"Simple Error Handler.vi"("error in (no error)"=w205) -> ()  [unwired: 4 in, 5 out]
    }
  }
